vi "VI Tree.vi"   [LabVIEW 2013, in "Agilent 3458.lvlib"]
doc: "This is the instrument driver for the AG 3458A. The VI Tree displays all the user-callable VIs of the instrument driver in an organized table."
uses:
  Agilent 3458.lvlib
  Data/Read Measurement(Single Point).vi
  Data/Low Level/Fetch Measurement(Single Point).vi
panel:
  # "© 2007 National Instruments.  ALL RIGHTS RESERVED."
  # "SEE DIAGRAM\nFOR VI TREE."
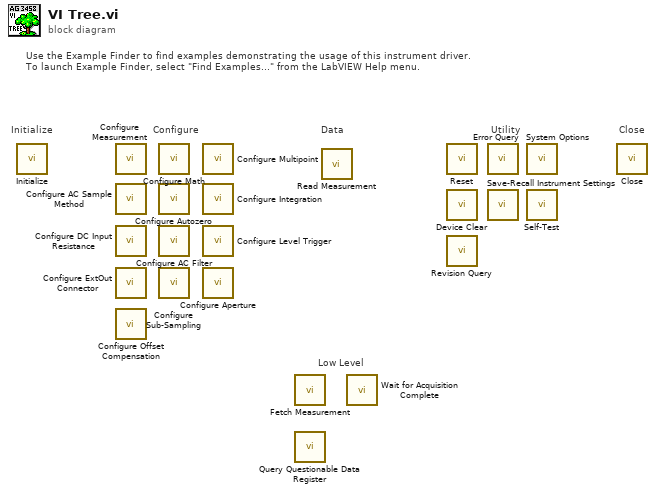
[diagram p0: block diagram]
diagram:
  # "Low Level"
  # "Use the Example Finder to find examples demonstrating the usage of this instrument driver.\nTo launch Example Finder, select \"Find Examples...\" from the LabVIEW Help menu."
  # "Configure"
  # "Utility"
  # "Data"
  # "Close"
  # "Initialize"
  n1 = call "Initialize.vi"() -> ()  [unwired: 10 in, 2 out]
  n2 = call "Configure Measurement.vi"() -> ()  [unwired: 14 in, 2 out]
  n3 = call "Configure AC Sample Method.vi"() -> ()  [unwired: 10 in, 2 out]
  n4 = call "Configure DC Input Resistance.vi"() -> ()  [unwired: 10 in, 2 out]
  n5 = call "Configure ExtOut Connector.vi"() -> ()  [unwired: 10 in, 2 out]
  n6 = call "Configure Offset Compensation.vi"() -> ()  [unwired: 10 in, 2 out]
  n7 = call "Configure Math.vi"() -> ()  [unwired: 14 in, 2 out]
  n8 = call "Configure Autozero.vi"() -> ()  [unwired: 10 in, 2 out]
  n9 = call "Configure AC Filter.vi"() -> ()  [unwired: 10 in, 2 out]
  n10 = call "Configure Sub-Sampling.vi"() -> ()  [unwired: 10 in, 2 out]
  n11 = call "Configure Multipoint.vi"() -> ()  [unwired: 10 in, 2 out]
  n12 = call "Configure Integration.vi"() -> ()  [unwired: 10 in, 2 out]
  n13 = call "Configure Level Trigger.vi"() -> ()  [unwired: 10 in, 2 out]
  n14 = call "Configure Aperture.vi"() -> ()  [unwired: 10 in, 2 out]
  n15 = call-poly "Fetch Measurement.vi"() -> ()  [unwired: 13 in, 3 out]
  n16 = call "Query Questionable Data Register.vi"() -> ()  [unwired: 9 in, 3 out]
  n17 = call-poly "Read Measurement.vi"() -> ()  [unwired: 13 in, 3 out]
  n18 = call "Wait for Acquisition Complete.vi"() -> ()  [unwired: 10 in, 2 out]
  n19 = call "Reset.vi"() -> ()  [unwired: 10 in, 2 out]
  n20 = call "Device Clear.vi"() -> ()  [unwired: 10 in, 2 out]
  n21 = call "Revision Query.vi"() -> ()  [unwired: 7 in, 5 out]
  n22 = call "Error Query.vi"() -> ()  [unwired: 8 in, 4 out]
  n23 = call "Save-Recall Instrument Settings.vi"() -> ()  [unwired: 10 in, 2 out]
  n24 = call "System Options.vi"() -> ()  [unwired: 10 in, 2 out]
  n25 = call "Self-Test.vi"() -> ()  [unwired: 10 in, 2 out]
  n26 = call "Close.vi"() -> ()  [unwired: 11 in, 1 out]
